vi "Test General each Comand Response.vi"(8 "error in (no error)":errorcluster, 11 "TestCase in":refnum<class "tests_actions.lvclass">) -> (0 "error out":errorcluster, 3 "TestCase out":refnum<class "tests_actions.lvclass">)   [LabVIEW 2019, in "tests_actions.lvclass"]
doc: "Test of each command of simulated commands and their respective responses"
uses:
  tests_actions.lvclass
  Clases Hijos/Simulated/Simulated uC.lvclass
  <vilib>/addons/_JKI Toolkits/VI Tester/TestCase.llb/TestCase.lvclass
  C:/Program Files/National Instruments/LabVIEW 2019/vi.lib/addons/_JKI Toolkits/VI Tester/TestCase.llb/TestCase.lvclass
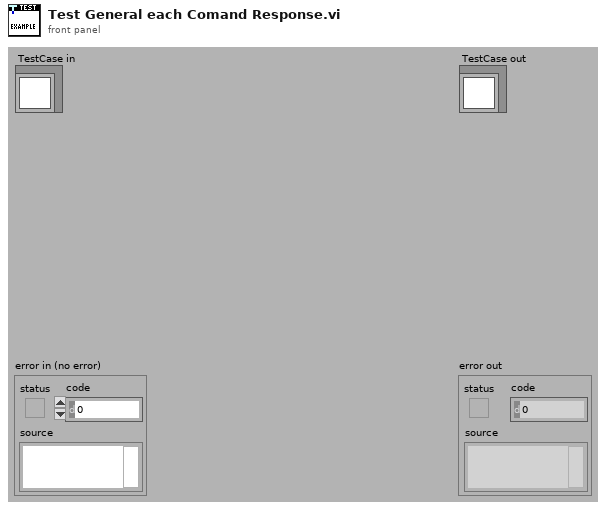
[diagram p1: front panel]
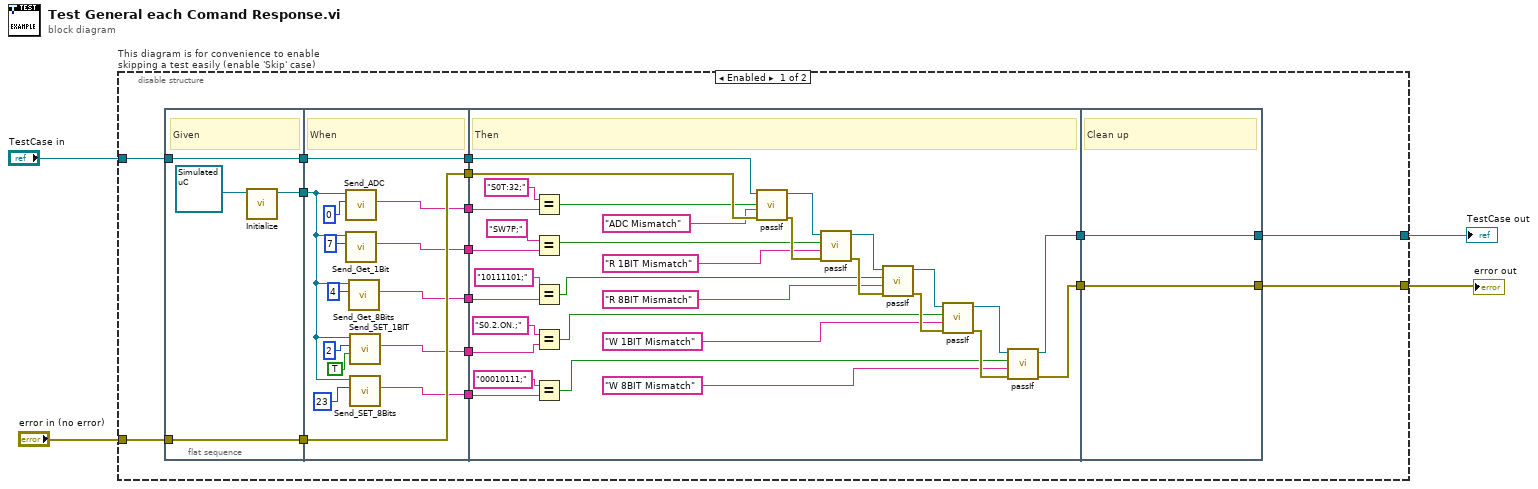
[diagram p0: block diagram]
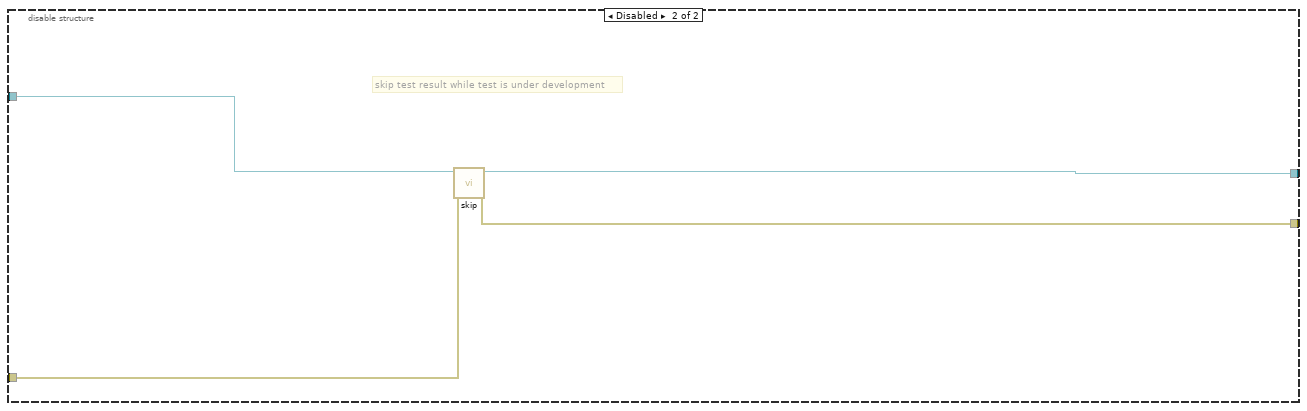
[diagram p2: hidden frame]
diagram:
  n1 = disable-structure "This diagram is for convenience to enable skipping a test easily (enable 'Skip' case)" shown="Enabled" {
    disable-tunnel: "TestCase in" -> [w15 w76]
    disable-tunnel: [w6 w74] -> w1
    disable-tunnel: [w5 w75] -> w3
    disable-tunnel: "error in (no error)" -> [w19 w73]
    frame Enabled {
      n2 = flat-sequence {
        tunnel: w19 -> [w24]
        tunnel: [w24] -> w18
        tunnel: w15 -> [w23]
        tunnel: [w23] -> w17
        tunnel: [w21] -> w14
        tunnel: [w38] -> w20
        tunnel: w18 -> [w38]
        tunnel: w17 -> [w37]
        tunnel: [w37] -> w16
        tunnel: w14 -> [w36]
        tunnel: [w29] -> w13
        tunnel: [w28] -> w12
        tunnel: [w27] -> w11
        tunnel: [w26] -> w10
        tunnel: [w25] -> w9
        tunnel: w20 -> [w54]
        tunnel: w16 -> [w60]
        tunnel: w13 -> [w70]
        tunnel: w12 -> [w67]
        tunnel: w11 -> [w61]
        tunnel: w10 -> [w62]
        tunnel: w9 -> [w63]
        tunnel: [w55] -> w8
        tunnel: [w49] -> w7
        tunnel: w8 -> [w72]
        tunnel: w7 -> [w71]
        tunnel: [w72] -> w6
        tunnel: [w71] -> w5
        frame #0 {
          # "Given"
          n3 = call-dynamic "Initialize.vi"("Simulated uC in"=refnum<class "Simulated uC.lvclass"> refnum ("Simulated uC.lvclass")) -> ("Simulated uC out"=w21:refnum<class "Simulated uC.lvclass">)  [unwired: 9 in, 1 out]
        }
        frame #1 {
          # "When"
          n4 = call-dynamic "Send_ADC.vi"("Channel"=u8 0, "Simulated uC in"=w36) -> ("Expected Response"=w29:string)  [unwired: 7 in, 2 out]
          n5 = call-dynamic "Send_Get_1Bit.vi"("Channel"=u8 7, "Simulated uC in"=w36) -> ("Response"=w28:string)  [unwired: 7 in, 2 out]
          n6 = call-dynamic "Send_Get_8Bits.vi"("Channel"=u8 4, "Simulated uC in"=w36) -> ("Response"=w27:string)  [unwired: 7 in, 2 out]
          n7 = call-dynamic "Send_SET_1BIT.vi"("Encender?"=TRUE, "Channel"=u8 2, "Simulated uC in"=w36) -> ("Response"=w26:string)  [unwired: 6 in, 2 out]
          n8 = call-dynamic "Send_SET_8Bits.vi"("Valor8 bits"=u8 23, "Simulated uC in"=w36) -> ("Response"=w25:string)  [unwired: 7 in, 2 out]
        }
        frame #2 {
          # "Then"
          n9 = Equal?(x="S0T:32;", y=w70) -> (x = y?=w48:bool)
          n10 = Equal?(x="SW7P;", y=w67) -> (x = y?=w47:bool)
          n11 = Equal?(x="10111101;", y=w61) -> (x = y?=w46:bool)
          n12 = Equal?(x="S0.2.ON.;", y=w62) -> (x = y?=w45:bool)
          n13 = Equal?(x="00010111;", y=w63) -> (x = y?=w44:bool)
          n14 = call-dynamic "passIf.vi"("error in (no error)"=w54, "message (\"\")"="ADC Mismatch" ("message (\"\")"), "pass"=w48, "TestCase in"=w60) -> ("error out"=w53:errorcluster, "TestCase out"=w59:refnum<class "tests_actions.lvclass">)  [unwired: 6 in]
          n15 = call-dynamic "passIf.vi"("error in (no error)"=w53, "message (\"\")"="R 1BIT Mismatch" ("message (\"\")"), "pass"=w47, "TestCase in"=w59) -> ("error out"=w52:errorcluster, "TestCase out"=w58:refnum<class "tests_actions.lvclass">)  [unwired: 6 in]
          n16 = call-dynamic "passIf.vi"("error in (no error)"=w52, "message (\"\")"="R 8BIT Mismatch" ("message (\"\")"), "pass"=w46, "TestCase in"=w58) -> ("error out"=w51:errorcluster, "TestCase out"=w57:refnum<class "tests_actions.lvclass">)  [unwired: 6 in]
          n17 = call-dynamic "passIf.vi"("error in (no error)"=w51, "message (\"\")"="W 1BIT Mismatch" ("message (\"\")"), "pass"=w45, "TestCase in"=w57) -> ("error out"=w50:errorcluster, "TestCase out"=w56:refnum<class "tests_actions.lvclass">)  [unwired: 6 in]
          n18 = call-dynamic "passIf.vi"("error in (no error)"=w50, "message (\"\")"="W 8BIT Mismatch" ("message (\"\")"), "pass"=w44, "TestCase in"=w56) -> ("error out"=w49:errorcluster, "TestCase out"=w55:refnum<class "tests_actions.lvclass">)  [unwired: 6 in]
        }
        frame #3 {
          # "Clean up"
        }
      }
    }
    frame Disabled {
      # "skip test result while test is under development"
      n19 = call <vilib>:"skip.vi"("error in (no error)"=w73, "TestCase in"=w76) -> ("error out"=w75:errorcluster, "TestCase out"=w74:refnum<class "tests_actions.lvclass">)  [unwired: 8 in]
    }
  }
  "error out" <- w3
  "TestCase out" <- w1
